vi "FPGAExample.vi"() -> ()   [LabVIEW 2016]
uses:
  <vilib>/rvi/Emulation/niFpgaGetClockAttributes.vi
  <vilib>/rvi/Emulation/niFpgaSctlEmulationGetInTimedLoop.vi
  <vilib>/rvi/Emulation/niFpgaEmulationReportErrorSimple.vi
  <vilib>/rvi/Emulation/niFpgaCriticalErrorInLSC.vi
  <vilib>/rvi/interface/RandomDataEmulation/niFpgaRandomDataHandleErrors.vi
  <vilib>/rvi/DataTransferAndStorage/Container/XNode/niFpgaContainer.xnode
  <vilib>/rvi/interface/RandomDataEmulation/nirviRandomDataFpgaReadWriteTemplate.vi
panel:
  out "My Array Indicator":u64[](array[numeric])
  in  "My Array Control":u64[](array[numeric])=[0, 0, 0, 0, 0]
  out "IRQ Loop Count":i32
  out "My Indicator":u64
  in  "My Control":u64
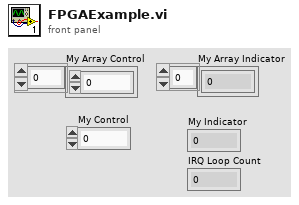
[diagram p1: front panel]
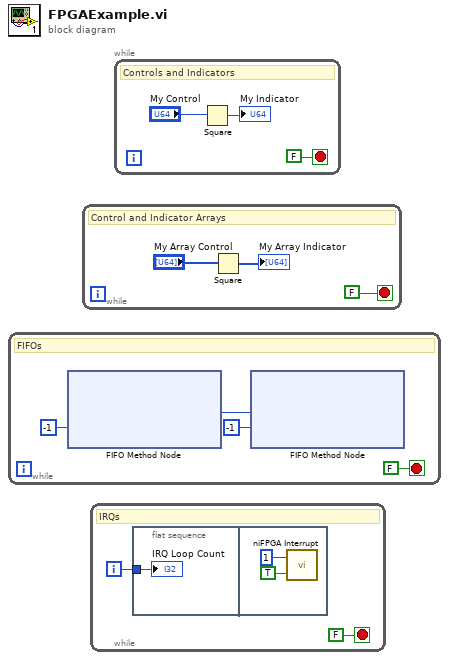
[diagram p0: block diagram]
diagram:
  n1 = while {
    stop <- FALSE stop-if-true
    # "FIFOs"
    n2 = xnode ("FIFO Method Node")("Timeout"=-1) -> ("Element"=w3:u32)  [unwired: 1 in, 2 out]
    n3 = xnode ("FIFO Method Node")("Element"=w3, "Timeout"=-1) -> ()  [unwired: 1 in, 2 out]
  }
  n4 = while {
    stop <- FALSE stop-if-true
    # "Control and Indicator Arrays"
    n5 = Square(x="My Array Control") -> (x^2=→"My Array Indicator":u64[])
  }
  n6 = while {
    i -> [w8]
    stop <- FALSE stop-if-true
    # "IRQs"
    n7 = flat-sequence {
      tunnel: w8 -> [w10]
      frame #0 {
        "IRQ Loop Count" <- w10
      }
      frame #1 {
        n8 = call <vilib>:"niFPGA Interrupt.vi"("Wait Until Cleared (F)"=TRUE, "IRQ Number (0)"=u8 1) -> ()  [unwired: 1 in]
      }
    }
  }
  n9 = while {
    stop <- FALSE stop-if-true
    # "Controls and Indicators"
    n10 = Square(x="My Control") -> (x^2=→"My Indicator":u64)
  }
